vi "Main.vi"() -> ()   [LabVIEW 2014]
uses:
  patiant and daq params.ctl
  CMD Report enum.ctl
  CMD DA enum.ctl
  CMD LOG enum.ctl
  CMD DAQ enum.ctl
  CMD UI enum.ctl
  set_get.ctl
  set-get-size.ctl
panel:
  in  "Tab Control":enum32{"Settings", "Data / Run"}(tab)=enum."Data / Run"
  in  "The Cluster":T1={"DAQ Parameters"={"Sampling rate"=600.0, "Max_volt"=10.0, "Min_volt"=-10.0, "DAQmx Physical Channels \nHR,SC"="Dev2/ai0:1", "Resting State"=TRUE, "Analyze every (s)"=3.755869993686643}, "Patient Info \n(Updates automatically when reading from file)"={"Patient Name"="ploni almoni", "Patient ID"="1234567", "Patient Age"=20.0, "Gender"="Female"}, "Raw Data Read Path"=path "", "Avg HR "=60.0, "Avg SC  "=3.0} {"DAQ Parameters"."Analyze every (s)" min=0.01 max=10.0 scale=0.0..10.0; "DAQ Parameters"."Min_volt" scale=-10.0..10.0; "DAQ Parameters"."Max_volt" scale=0.0..10.0}
  in  "Read from file":bool
  out "current SC":dbl
  out "current HR":dbl
  out "Both Parameters over threshold":bool
  out "SC over Threshold":bool
  out "HR over threshold":bool
  out "Skin Conductance":dbl[](graph)
  out "HR":dbl[](graph)
  in  "Create Report":bool
  in  "EXIT":bool
  in  "RECORD":bool
  in  "Start/Stop DAQ":bool
  out "Arterial Pressure (Raw Data)":dbl[](graph)
  out "Skin Conductance (Raw Data)":dbl[](graph)
  # "Read from card"
  # "Leave zero if unkown \nand run in Resting mode first"
  # "Active State"
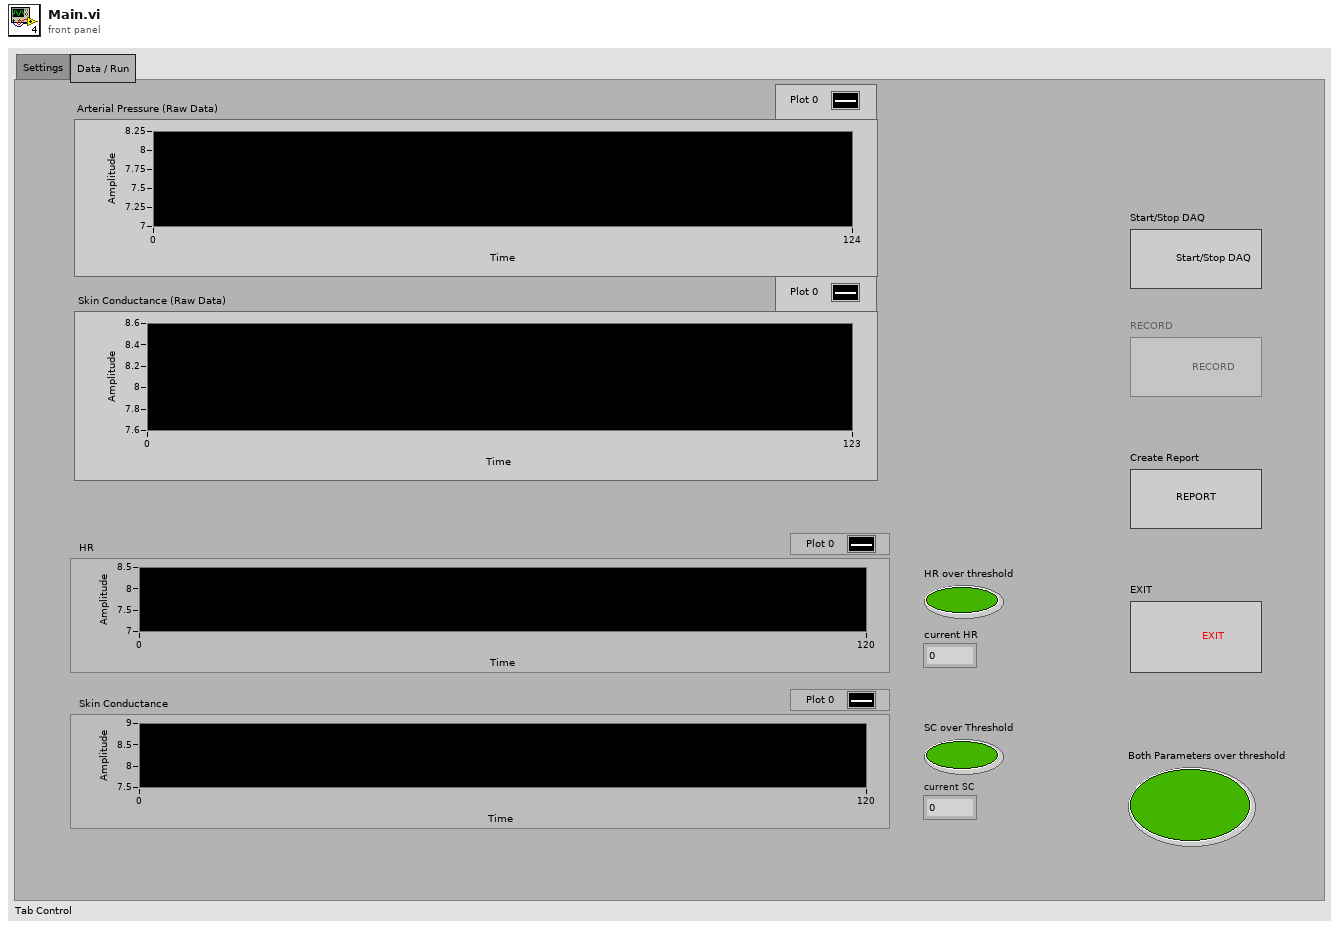
[diagram p1: front panel]
types:
  T1 = typedef "patiant and daq params.ctl" = cluster{"DAQ Parameters":cluster{"Sampling rate":dbl, "Max_volt":dbl, "Min_volt":dbl, "DAQmx Physical Channels \nHR,SC":tag, "Resting State":bool, "Analyze every (s)":dbl}, "Patient Info \n(Updates automatically when reading from file)":cluster{"Patient Name":string, "Patient ID":string, "Patient Age":dbl, "Gender":string}, "Raw Data Read Path":path, "Avg HR ":dbl, "Avg SC  ":dbl}
  T2 = typedef "CMD UI enum.ctl" = enum16{"Init all", "Update Patient Info", "Update Analyzed", "Create Report", "Analyze Data", "Start DAQ", "Start Read", "LOG Data", "Stop LOG Data", "Stop DAQ", "Stop Read", "EXIT"}
  T3 = typedef "CMD DAQ enum.ctl" = enum16{"Init DAQ", "Init Read From File", "DAQ", "Read From File", "Stop DAQ", "Stop Read From File", "Exit"}
  T4 = typedef "CMD LOG enum.ctl" = enum16{"Start Log", "Log", "Stop Log", "Exit"}
  T5 = typedef "CMD DA enum.ctl" = enum16{"Wait", "Analyze", "Meta Analyze", "Exit"}
  T6 = typedef "CMD Report enum.ctl" = enum16{"Create Report", "Exit"}
  T7 = cluster{"Start/Stop DAQ":refnum<vi>, "Create Report":refnum<vi>, "RECORD":refnum<vi>, "Read from file":refnum<vi>, "EXIT":refnum<vi>, "The Cluster":refnum<vi>}
  T8 = typedef "set_get.ctl" = enum16{"Set", "Get"}
  T9 = cluster{"CMD UI":refnum<queue>, "CMD REP":refnum<queue>, "CMD DA":refnum<queue>, "CMD DAQ":refnum<queue>, "CMD LOG":refnum<queue>, "Data LOG":refnum<queue>, "Data Display":refnum<queue>}
  T10 = typedef "set-get-size.ctl" = enum16{"set", "get", "size"}
  T11 = cluster{string, string, dbl, "Combo Box":string, dbl}
  T12 = cluster{"Boolean":bool, "Boolean":bool, bool, dbl, dbl}
  T13 = cluster{"The Cluster":T1, "Arterial Pressure (Raw Data)":refnum<vi>, "Skin Conductance (Raw Data)":refnum<vi>, "HR":refnum<vi>, "Skin Conductance":refnum<vi>}
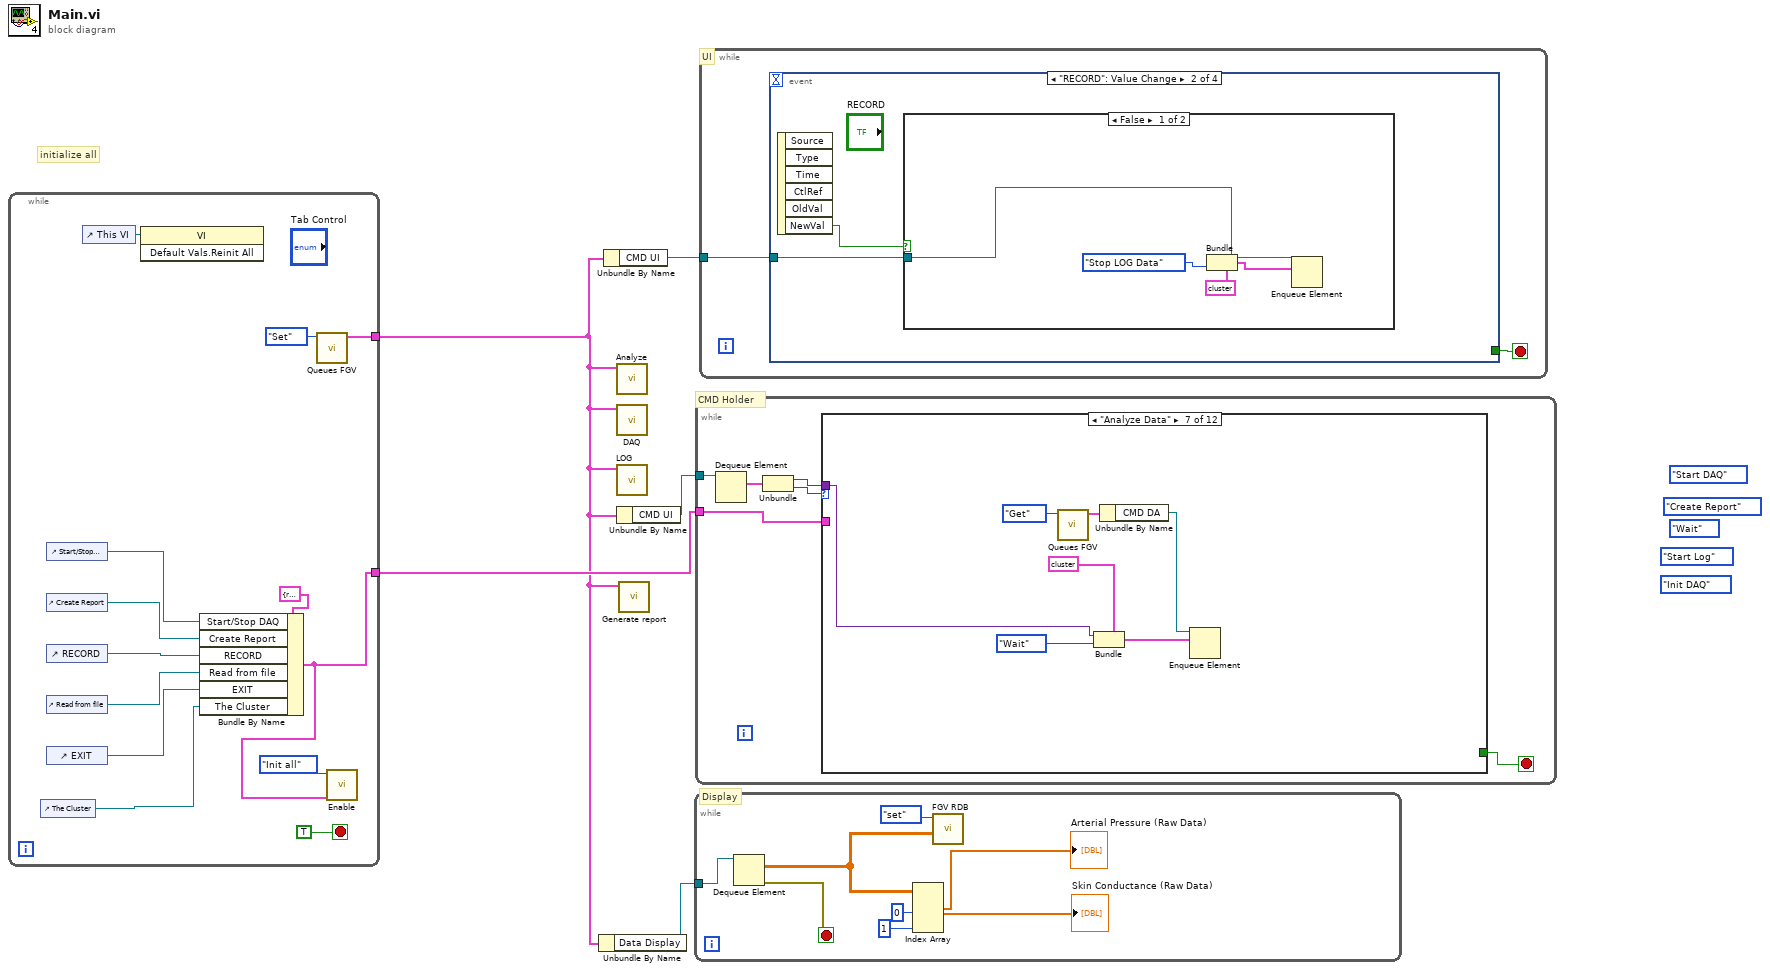
[diagram p0: block diagram]
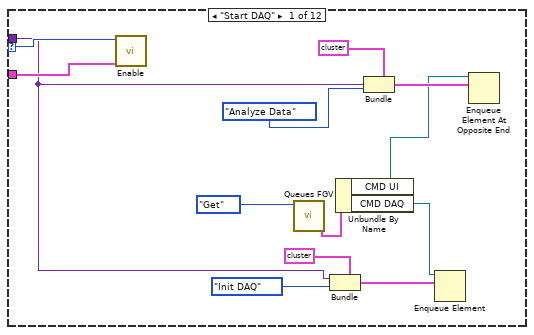
[diagram p2: hidden frame]
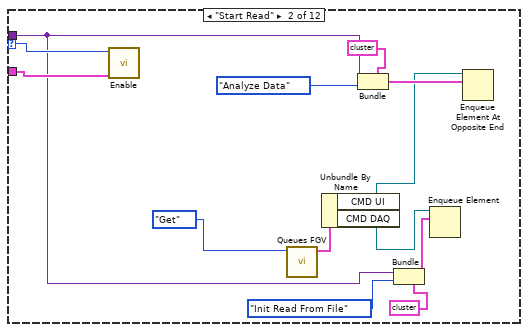
[diagram p3: hidden frame]
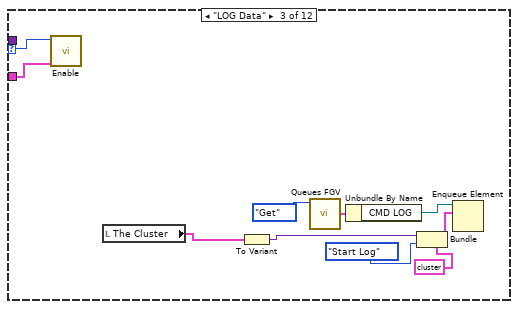
[diagram p4: hidden frame]
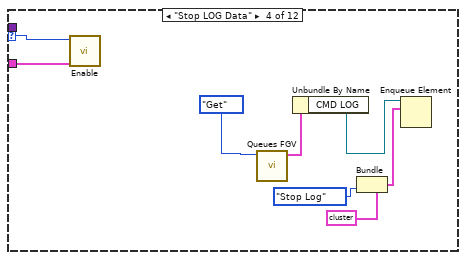
[diagram p5: hidden frame]
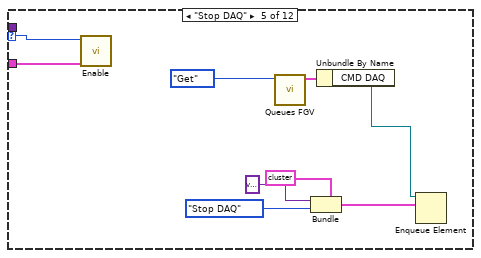
[diagram p6: hidden frame]
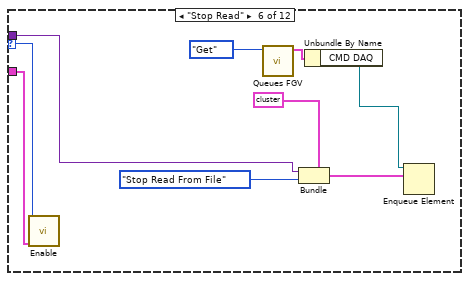
[diagram p7: hidden frame]
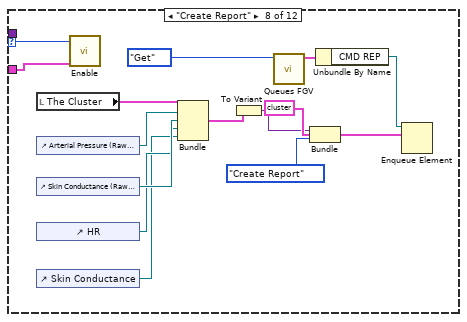
[diagram p8: hidden frame]
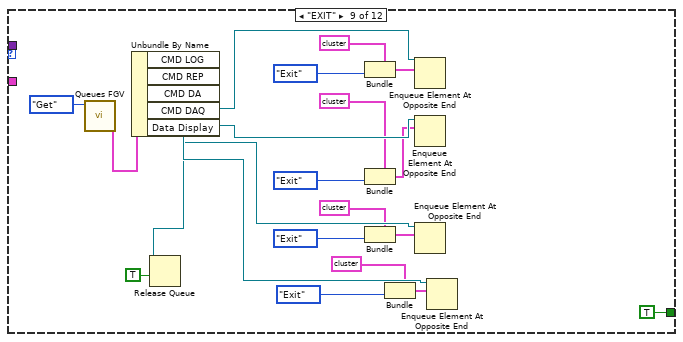
[diagram p9: hidden frame]
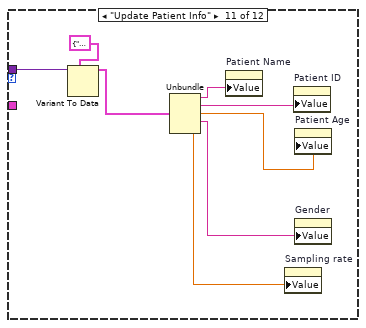
[diagram p11: hidden frame]
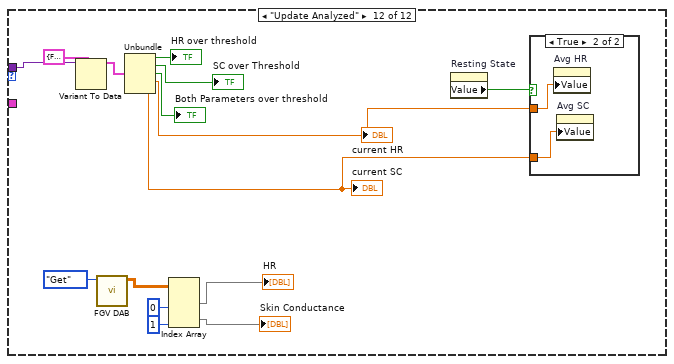
[diagram p12: hidden frame]
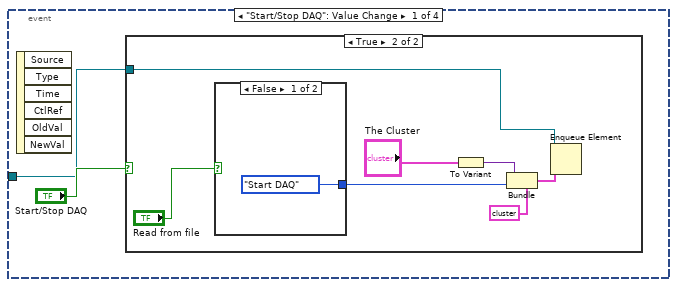
[diagram p14: hidden frame]
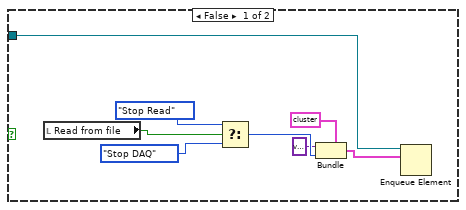
[diagram p15: hidden frame]
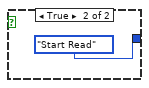
[diagram p16: hidden frame]
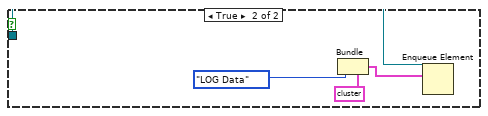
[diagram p17: hidden frame]
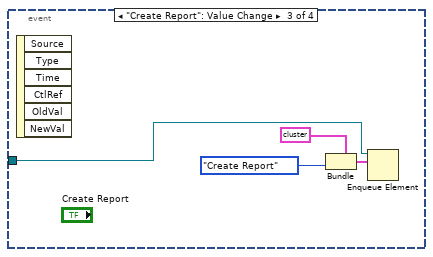
[diagram p18: hidden frame]
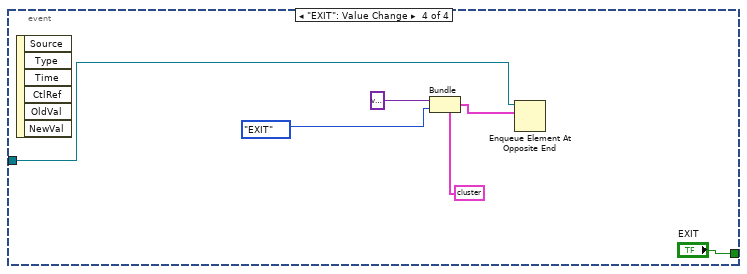
[diagram p19: hidden frame]
diagram:
  (unwired) CMD_UI_enum."Start DAQ"
  (unwired) CMD_DAQ_enum."Init DAQ"
  (unwired) CMD_LOG_enum."Start Log"
  (unwired) CMD_DA_enum."Wait"
  (unwired) CMD_Report_enum."Create Report"
  # "Display"
  # "CMD Holder"
  # "UI"
  # "initialize all"
  n1 = while {
    tunnel: [w6] -> w2
    tunnel: [w9] -> w1
    stop <- TRUE stop-if-true
    n2 = control-ref of="The Cluster"() -> (w7:refnum<vi>)
    n3 = control-ref of="Start/Stop DAQ"() -> (w12:refnum<vi>)
    n4 = control-ref of="Create Report"() -> (w13:refnum<vi>)
    n5 = control-ref of="RECORD"() -> (w14:refnum<vi>)
    n6 = control-ref of="Read from file"() -> (w15:refnum<vi>)
    n7 = control-ref of="EXIT"() -> (w16:refnum<vi>)
    n8 = control-ref of="This VI"() -> (w8:refnum<vi>)
    n9 = invoke class="VI" method="Default Vals.Reinit All"(reference=w8) -> ()  [unwired: 2 in, 3 out]
    n10 = Bundle By Name(cluster=T7 {"Start/Stop DAQ"=refnum, "Create Report"=refnum, "RECORD"=refnum, "Read from file"=refnum, "EXIT"=refnum, "The Cluster"=refnum} ("output cluster"), "Start/Stop DAQ"=w12, "Create Report"=w13, "RECORD"=w14, "Read from file"=w15, "EXIT"=w16, "The Cluster"=w7) -> (w6:T7)
    n11 = call "Queues FGV.vi"("Enum"=set_get."Set") -> ("Queues"=w9:T9)  [unwired: 10 in]
    n12 = call "Enable.vi"("output cluster"=w6, "Enum"=CMD_UI_enum."Init all") -> ()  [unwired: 10 in]
  }
  n13 = Unbundle By Name(w1) -> ("Data Display"=w5:refnum<queue>)
  n14 = Unbundle By Name(w1) -> ("CMD UI"=w4:refnum<queue>)
  n15 = call "Analyze.vi"("Queues"=w1) -> ()  [unwired: 11 in]
  n16 = call "DAQ.vi"("Queues"=w1) -> ()  [unwired: 9 in, 1 out]
  n17 = call "LOG.vi"("Queues"=w1) -> ()  [unwired: 10 in, 1 out]
  n18 = Unbundle By Name(w1) -> ("CMD UI"=w3:refnum<queue>)
  n19 = call "Generate report.vi"("Queues"=w1) -> ()  [unwired: 11 in]
  n20 = while {
    tunnel: w5 -> [w26]
    stop <- w25 stop-if-true
    n21 = Dequeue Element(queue=w26) -> (element=w19:dbl[][], error out=w25:errorcluster)  [unwired: 2 in, 2 out]
    n22 = Index Array(array=w19, index (col) #1=0 ("disabled index (col)"), index (col) #2=1 ("index (col)")) -> (element #1=→"Arterial Pressure (Raw Data)":dbl[], element #2=→"Skin Conductance (Raw Data)":dbl[])  [unwired: 2 in]
    n23 = call "FGV RDB.vi"("Raw data in"=w19, "Command"=set-get-size."set" ("Enum")) -> ()  [unwired: 8 in, 2 out]
  }
  n24 = while {
    tunnel: w3 -> [w30]
    tunnel: w2 -> [w28]
    stop <- w27 stop-if-true
    n25 = Dequeue Element(queue=w30) -> (element=w32:cluster{variant, T2})  [unwired: 2 in, 3 out]
    n26 = Unbundle(w32) -> (w29:variant, w31:T2)
    n27 = case shown="\"Analyze Data\"" w31 {
      selector: w31 -> [w39 w52 w62 w70 w80 w87 _ w110 _ _ _ _]
      tunnel: w29 -> [w33 w46 _ _ _ w88 w95 _ _ _ w145 w160]
      tunnel: w28 -> [w34 w47 w59 w69 w77 w86 _ w109 _ _ _ _]
      tunnel: [_ _ _ _ _ _ _ _ TRUE _ _ _] -> w27
      frame "Start DAQ" {
        n28 = call "Enable.vi"("output cluster"=w34, "Enum"=w39) -> ()  [unwired: 10 in]
        n29 = call "Queues FGV.vi"("Enum"=set_get."Get") -> ("Queues"=w44:T9)  [unwired: 10 in]
        n30 = Bundle(cluster=cluster{variant, T3} {variant, enum."Init DAQ"}, w33, CMD_DAQ_enum."Init DAQ") -> (w40:cluster{variant, T3})
        n31 = Unbundle By Name(w44) -> ("CMD UI"=w35:refnum<queue>, "CMD DAQ"=w43:refnum<queue>)
        n32 = Bundle(cluster=cluster{variant, T2} {variant, enum."Start DAQ"}, w33, CMD_UI_enum."Analyze Data") -> (w37:cluster{variant, T2})
        n33 = Enqueue Element(queue=w43, element=w40) -> ()  [unwired: 2 in, 3 out]
        n34 = Enqueue Element At Opposite End(queue=w35, element=w37) -> ()  [unwired: 2 in, 3 out]
      }
      frame "Start Read" {
        n35 = call "Enable.vi"("output cluster"=w47, "Enum"=w52) -> ()  [unwired: 10 in]
        n36 = call "Queues FGV.vi"("Enum"=set_get."Get") -> ("Queues"=w57:T9)  [unwired: 10 in]
        n37 = Unbundle By Name(w57) -> ("CMD UI"=w48:refnum<queue>, "CMD DAQ"=w56:refnum<queue>)
        n38 = Bundle(cluster=cluster{variant, T2} {variant, enum."Start DAQ"}, w46, CMD_UI_enum."Analyze Data") -> (w51:cluster{variant, T2})
        n39 = Bundle(cluster=cluster{variant, T3} {variant, enum."Init DAQ"}, w46, CMD_DAQ_enum."Init Read From File") -> (w53:cluster{variant, T3})
        n40 = Enqueue Element(queue=w56, element=w53) -> ()  [unwired: 2 in, 3 out]
        n41 = Enqueue Element At Opposite End(queue=w48, element=w51) -> ()  [unwired: 2 in, 3 out]
      }
      frame "LOG Data" {
        n42 = call "Enable.vi"("output cluster"=w59, "Enum"=w62) -> ()  [unwired: 10 in]
        n43 = local read "The Cluster"() -> (w61:T1)
        n44 = To Variant(anything=w61) -> (Variant=w60:variant)
        n45 = call "Queues FGV.vi"("Enum"=set_get."Get") -> ("Queues"=w67:T9)  [unwired: 10 in]
        n46 = Unbundle By Name(w67) -> ("CMD LOG"=w66:refnum<queue>)
        n47 = Bundle(cluster=cluster{variant, T4} {variant, enum."Start Log"}, w60, CMD_LOG_enum."Start Log") -> (w64:cluster{variant, T4})
        n48 = Enqueue Element(queue=w66, element=w64) -> ()  [unwired: 2 in, 3 out]
      }
      frame "Stop LOG Data" {
        n49 = call "Enable.vi"("output cluster"=w69, "Enum"=w70) -> ()  [unwired: 10 in]
        n50 = call "Queues FGV.vi"("Enum"=set_get."Get") -> ("Queues"=w75:T9)  [unwired: 10 in]
        n51 = Unbundle By Name(w75) -> ("CMD LOG"=w74:refnum<queue>)
        n52 = Bundle(cluster=cluster{variant, T4} {variant, enum."Start Log"}, CMD_LOG_enum."Stop Log") -> (w72:cluster{variant, T4})  [unwired: 1 in]
        n53 = Enqueue Element(queue=w74, element=w72) -> ()  [unwired: 2 in, 3 out]
      }
      frame "Stop DAQ" {
        n54 = call "Enable.vi"("output cluster"=w77, "Enum"=w80) -> ()  [unwired: 10 in]
        n55 = call "Queues FGV.vi"("Enum"=set_get."Get") -> ("Queues"=w84:T9)  [unwired: 10 in]
        n56 = Bundle(cluster=cluster{variant, T3} {variant, enum."Init DAQ"}, variant, CMD_DAQ_enum."Stop DAQ") -> (w81:cluster{variant, T3})
        n57 = Unbundle By Name(w84) -> ("CMD DAQ"=w83:refnum<queue>)
        n58 = Enqueue Element(queue=w83, element=w81) -> ()  [unwired: 2 in, 3 out]
      }
      frame "Stop Read" {
        n59 = call "Enable.vi"("output cluster"=w86, "Enum"=w87) -> ()  [unwired: 10 in]
        n60 = call "Queues FGV.vi"("Enum"=set_get."Get") -> ("Queues"=w93:T9)  [unwired: 10 in]
        n61 = Bundle(cluster=cluster{variant, T3} {variant, enum."Init DAQ"}, w88, CMD_DAQ_enum."Stop Read From File") -> (w89:cluster{variant, T3})
        n62 = Unbundle By Name(w93) -> ("CMD DAQ"=w92:refnum<queue>)
        n63 = Enqueue Element(queue=w92, element=w89) -> ()  [unwired: 2 in, 3 out]
      }
      frame "Analyze Data" {
        n64 = call "Queues FGV.vi"("Enum"=set_get."Get") -> ("Queues"=w98:T9)  [unwired: 10 in]
        n65 = Bundle(cluster=cluster{variant, T5} {variant, enum."Wait"}, w95, CMD_DA_enum."Wait") -> (w101:cluster{variant, T5})
        n66 = Unbundle By Name(w98) -> ("CMD DA"=w99:refnum<queue>)
        n67 = Enqueue Element(queue=w99, element=w101) -> ()  [unwired: 2 in, 3 out]
      }
      frame "Create Report" {
        n68 = local read "The Cluster"() -> (w106:T1)
        n69 = control-ref of="Arterial Pressure (Raw Data)"() -> (w105:refnum<vi>)
        n70 = control-ref of="Skin Conductance (Raw Data)"() -> (w104:refnum<vi>)
        n71 = control-ref of="HR"() -> (w103:refnum<vi>)
        n72 = control-ref of="Skin Conductance"() -> (w102:refnum<vi>)
        n73 = call "Enable.vi"("output cluster"=w109, "Enum"=w110) -> ()  [unwired: 10 in]
        n74 = Bundle("The Cluster"=w106, "Arterial Pressure (Raw Data)"=w105, "Skin Conductance (Raw Data)"=w104, "HR"=w103, "Skin Conductance"=w102) -> (w107:T13)  [unwired: 1 in]
        n75 = To Variant(anything=w107) -> (Variant=w108:variant)
        n76 = call "Queues FGV.vi"("Enum"=set_get."Get") -> ("Queues"=w113:T9)  [unwired: 10 in]
        n77 = Bundle(cluster=cluster{variant, T6} {variant, enum."Create Report"}, w108, CMD_Report_enum."Create Report") -> (w116:cluster{variant, T6})
        n78 = Unbundle By Name(w113) -> ("CMD REP"=w114:refnum<queue>)
        n79 = Enqueue Element(queue=w114, element=w116) -> ()  [unwired: 2 in, 3 out]
      }
      frame "EXIT" {
        n80 = call "Queues FGV.vi"("Enum"=set_get."Get") -> ("Queues"=w136:T9)  [unwired: 10 in]
        n81 = Unbundle By Name(w136) -> ("CMD LOG"=w131:refnum<queue>, "CMD REP"=w130:refnum<queue>, "CMD DA"=w129:refnum<queue>, "CMD DAQ"=w135:refnum<queue>, "Data Display"=w119:refnum<queue>)
        n82 = Release Queue(queue=w119, force destroy? (F)=TRUE) -> ()  [unwired: 1 in, 3 out]
        n83 = Bundle(cluster=cluster{variant, T4} {variant, enum."Start Log"}, CMD_LOG_enum."Exit") -> (w126:cluster{variant, T4})  [unwired: 1 in]
        n84 = Bundle(cluster=cluster{variant, T6} {variant, enum."Create Report"}, CMD_Report_enum."Exit") -> (w123:cluster{variant, T6})  [unwired: 1 in]
        n85 = Bundle(cluster=cluster{variant, T5} {variant, enum."Wait"}, CMD_DA_enum."Exit") -> (w120:cluster{variant, T5})  [unwired: 1 in]
        n86 = Bundle(cluster=cluster{variant, T3} {variant, enum."Init DAQ"}, CMD_DAQ_enum."Exit") -> (w132:cluster{variant, T3})  [unwired: 1 in]
        n87 = Enqueue Element At Opposite End(queue=w131, element=w126) -> ()  [unwired: 2 in, 3 out]
        n88 = Enqueue Element At Opposite End(queue=w130, element=w123) -> ()  [unwired: 2 in, 3 out]
        n89 = Enqueue Element At Opposite End(queue=w129, element=w120) -> ()  [unwired: 2 in, 3 out]
        n90 = Enqueue Element At Opposite End(queue=w135, element=w132) -> ()  [unwired: 2 in, 3 out]
      }
      frame "Init all", Default {
      }
      frame "Update Patient Info" {
        n91 = Variant To Data(type=T11 {"", "", 0.0, "Combo Box"="", 0.0} ("output cluster"), Variant=w145) -> (data=w143:T11)  [unwired: 1 in, 1 out]
        n92 = Unbundle(w143) -> (w142:string, w141:string, w140:dbl, "Combo Box"=w139:string, w138:dbl)
        n93 = property on="Patient Name" class="Str"("Value"=w142) -> ()  [unwired: 2 in, 2 out]
        n94 = property on="Sampling rate" class="DigNum (strict)"("Value"=w138) -> ()  [unwired: 2 in, 2 out]
        n95 = property on="Patient ID" class="Str"("Value"=w141) -> ()  [unwired: 2 in, 2 out]
        n96 = property on="Patient Age" class="DigNum (strict)"("Value"=w140) -> ()  [unwired: 2 in, 2 out]
        n97 = property on="Gender" class="CmbBox"("Value"=w139) -> ()  [unwired: 2 in, 2 out]
      }
      frame "Update Analyzed" {
        n98 = Variant To Data(type=T12 {"Boolean"=FALSE, "Boolean"=TRUE, FALSE, 0.0, 0.0} ("output cluster"), Variant=w160) -> (data=w158:T12)  [unwired: 1 in, 1 out]
        n99 = call "FGV DAB.vi"("Enum"=set_get."Get") -> ("DAB"=w153:dbl[][])  [unwired: 10 in]
        n100 = Unbundle(w158) -> ("Boolean"=→"HR over threshold":bool, "Boolean"=→"SC over Threshold":bool, →"Both Parameters over threshold":bool, w148:dbl, w147:dbl)
        "current HR" <- w148
        "current SC" <- w147
        n101 = Index Array(array=w153, index (col) #1=0 ("disabled index (col)"), index (col) #2=1 ("index (col)")) -> (element #1=→"HR":dbl[], element #2=→"Skin Conductance":dbl[])  [unwired: 2 in]
        n102 = property on="Resting State" class="Bool (strict)"() -> ("Value"=w146:bool)  [unwired: 2 in, 2 out]
        n103 = case shown="True" w146 {
          tunnel: w148 -> [_ w162]
          tunnel: w147 -> [_ w161]
          frame False {
          }
          frame True {
            n104 = property on="Avg HR" class="DigNum (strict)"("Value"=w162) -> ()  [unwired: 2 in, 2 out]
            n105 = property on="Avg SC" class="DigNum (strict)"("Value"=w161) -> ()  [unwired: 2 in, 2 out]
          }
        }
      }
    }
  }
  n106 = while {
    tunnel: w4 -> [w164]
    stop <- w163 stop-if-true
    n107 = event shown="[1] \"RECORD\": Value Change" {
      selector: _ -> [_ _ _ _]
      dyn-events: _ -> [_ _ _ _]
      timeout: _ -> [_ _ _ _]
      tunnel: w164 -> [w165 w184 w195 w200]
      tunnel: [_ _ _ "EXIT"] -> w163
      event "Start/Stop DAQ": Value Change {
        n108 = event-data() -> ()  [unwired: 1 in, 6 out]
        n109 = case shown="True" "Start/Stop DAQ" {
          tunnel: w165 -> [w173 w181]
          frame False {
            n110 = local read "Read from file"() -> (w169:bool)
            n111 = Select(t=CMD_UI_enum."Stop Read", s=w169, f=CMD_UI_enum."Stop DAQ") -> (s? t:f=w168:T2)
            n112 = Bundle(cluster=cluster{variant, T2} {variant, enum."Start DAQ"}, variant, w168) -> (w174:cluster{variant, T2})
            n113 = Enqueue Element(queue=w173, element=w174) -> ()  [unwired: 2 in, 3 out]
          }
          frame True {
            n114 = case shown="False" "Read from file" {
              tunnel: [CMD_UI_enum."Start DAQ" CMD_UI_enum."Start Read"] -> w178
              frame False {
              }
              frame True {
              }
            }
            n115 = To Variant(anything="The Cluster") -> (Variant=w176:variant)
            n116 = Bundle(cluster=cluster{variant, T2} {variant, enum."Start DAQ"}, w176, w178) -> (w179:cluster{variant, T2})
            n117 = Enqueue Element(queue=w181, element=w179) -> ()  [unwired: 2 in, 3 out]
          }
        }
      }
      event "RECORD": Value Change {
        n118 = event-data() -> ("NewVal"=w185:bool)  [unwired: 1 in, 5 out]
        n119 = case shown="False" w185 {
          tunnel: w184 -> [w187 w193]
          frame False {
            n120 = Bundle(cluster=cluster{variant, T2} {variant, enum."Start DAQ"}, CMD_UI_enum."Stop LOG Data") -> (w189:cluster{variant, T2})  [unwired: 1 in]
            n121 = Enqueue Element(queue=w187, element=w189) -> ()  [unwired: 2 in, 3 out]
          }
          frame True {
            n122 = Bundle(cluster=cluster{variant, T2} {variant, enum."Start DAQ"}, CMD_UI_enum."LOG Data") -> (w191:cluster{variant, T2})  [unwired: 1 in]
            n123 = Enqueue Element(queue=w193, element=w191) -> ()  [unwired: 2 in, 3 out]
          }
        }
      }
      event "Create Report": Value Change {
        n124 = event-data() -> ()  [unwired: 1 in, 6 out]
        n125 = Bundle(cluster=cluster{variant, T2} {variant, enum."Start DAQ"}, CMD_UI_enum."Create Report") -> (w197:cluster{variant, T2})  [unwired: 1 in]
        n126 = Enqueue Element(queue=w195, element=w197) -> ()  [unwired: 2 in, 3 out]
      }
      event "EXIT": Value Change {
        n127 = event-data() -> ()  [unwired: 1 in, 6 out]
        n128 = Bundle(cluster=cluster{variant, T2} {variant, enum."Start DAQ"}, variant, CMD_UI_enum."EXIT") -> (w203:cluster{variant, T2})
        n129 = Enqueue Element At Opposite End(queue=w200, element=w203) -> ()  [unwired: 2 in, 3 out]
      }
    }
  }
